vi "MoveMirror.vi"(1 "error in 2":errorcluster, 3 "POS X rad":dbl, 4 "POS Y rad":dbl) -> (0 "error out 2":errorcluster)   [LabVIEW 2013]
uses:
  Utilities/controls/ctlSeqFNs_PI_SysNr.ctl
  Variables/GlobalSetConfigurationPhysikalInstruments.vi
  Variables/GlobalSetNumberOfDigits_PhysikalInstruments.vi
  Variables/GlobalSetGetPositionParameters.vi
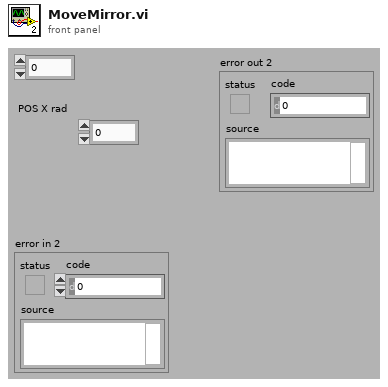
[diagram p1: front panel]
types:
  T1 = typedef "ctlSeqFNs_PI_SysNr.ctl" = enum16{"Zero", "E517", "E710"}
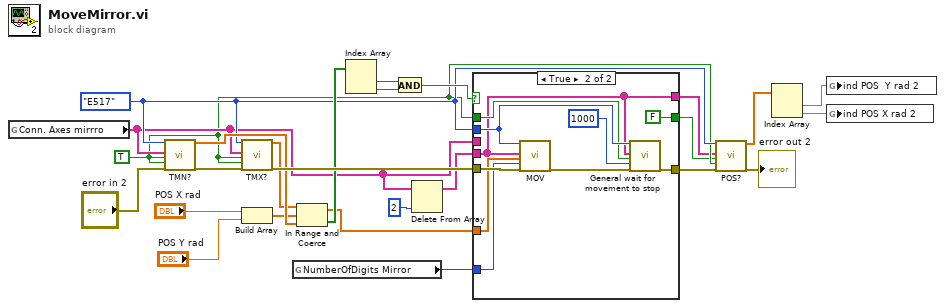
[diagram p0: block diagram]
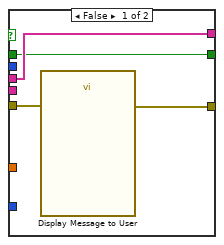
[diagram p2: hidden frame]
diagram:
  w5 = TRUE ("All axes?")
  w11 = ctlSeqFNs_PI_SysNr."E517" ("DeviceNr.")
  n1 = global read "GlobalSetConfigurationPhysikalInstruments.vi" "Conn. Axes mirrro"() -> (w7:string[])
  n2 = call "TMN?.vi"("System no."=w11, "Axes to query"=w7, "All axes?"=w5, "Axis identifier?"=w5, "error in"="error in 2") -> ("Minimum travel limit"=w22:dbl[], "error out"=w25:errorcluster)  [unwired: 13 in]
  n3 = call "TMX?.vi"("System no."=w11, "Axes to query"=w7, "All axes?"=w5, "Axis identifier?"=w5, "error in"=w25) -> ("Maximum travel limit"=w21:dbl[], "error out"=w24:errorcluster)  [unwired: 13 in]
  n4 = Build Array("POS X rad", "POS Y rad") -> (w20:dbl[])
  n5 = global read "GlobalSetNumberOfDigits_PhysikalInstruments.vi" "NumberOfDigits Mirror"() -> (w23:i32)
  n6 = In Range and Coerce(upper limit=w21, x=w20, lower limit=w22) -> (coerced(x)=w15:dbl[], In Range?=w19:bool[])
  n7 = Index Array(array=w19) -> (element #1=w18:bool, element #2=w17:bool)  [unwired: 2 in]
  n8 = And(x=w18, y=w17) -> (x .and. y?=w16:bool)
  n9 = Delete From Array(array=w7, index=2) -> (array with subset deleted=w8:string[])  [unwired: 1 in, 1 out]
  n10 = case shown="True" w16 {
    tunnel: w15 -> [_ w34]
    tunnel: w24 -> [w29 w40]
    tunnel: [w30 w38] -> w10
    tunnel: w8 -> [_ w32]
    tunnel: w11 -> [_ w37]
    tunnel: w23 -> [_ w35]
    tunnel: w7 -> [w28 _]
    tunnel: w5 -> [w27 w33]
    tunnel: [w28 w32] -> w4
    tunnel: [w27 FALSE] -> w3
    frame False {
      n11 = call "Display Message to User"("error in (no error)"=w29) -> ("error out"=w30:errorcluster)  [unwired: 9 in, 1 out]
    }
    frame True {
      n12 = call "MOV.vi"("System no."=w37, "Axes to move"=w32, "Position values"=w34, "No.of digits"=w35, "error in"=w40) -> ("error out"=w39:errorcluster)  [unwired: 14 in]
      n13 = call "General wait for movement to stop.vi"("System no."=w37, "Axes to wait for"=w32, "All axes?"=w33, "Additional wait time, ms"=u32 1000, "error in"=w39) -> ("error out"=w38:errorcluster)  [unwired: 13 in, 1 out]
    }
  }
  n14 = call "POS?.vi"("System no."=w11, "Axes to query"=w4, "All axes?"=w3, "Axis identifier?"=w5, "error in"=w10) -> ("Position"=w14:dbl[], "error out"=→"error out 2":errorcluster)  [unwired: 13 in]
  n15 = Index Array(array=w14) -> (element #1=w13:dbl, element #2=w12:dbl)  [unwired: 2 in]
  n16 = global write "GlobalSetGetPositionParameters.vi" "ind POS  Y rad 2"(w13) -> ()
  n17 = global write "GlobalSetGetPositionParameters.vi" "ind POS X rad 2"(w12) -> ()
